vi "nanomsg_pub.vi"() -> ()   [LabVIEW 2014]
uses:
  lvnanomsg/nanomsg_context.lvclass
  lvnanomsg/nanomsg_socket.lvclass
panel:
  out "loop":i32=1
  in  "port":i32=5555
  # "Nanomsg publisher VI"
  # "Launch multiple instances of this template VI on different ports, and use zmq_sub.vit to subscribe to them all simultaneously."
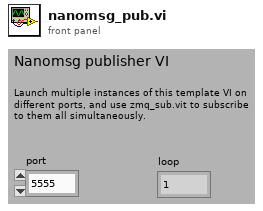
[diagram p1: front panel]
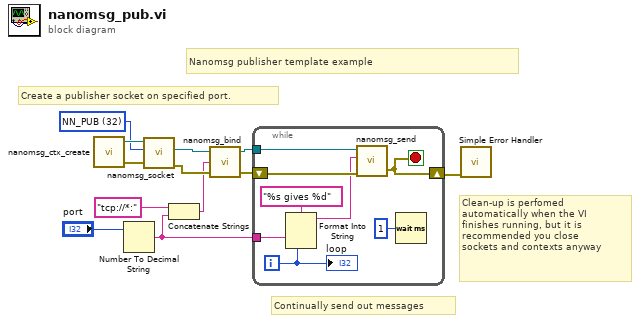
[diagram p0: block diagram]
diagram:
  w10 = 32 items=["NN_WS"=-4, "NN_TCP"=-3, "NN_IPC"=-2, "NN_INPROC"=-1, "NN_SOL_SOCKET"=0, "NN_PAIR"=16, "NN_PUB"=32, "NN_SUB"=33, "NN_REQ"=48, "NN_REP"=49, "NN_PUSH"=80, "NN_PULL"=81, "NN_SURVEYOR"=98, "NN_RESPONDENT"=99, "NN_BUS"=112] ("socket type")
  # "Clean-up is perfomed\nautomatically when the VI\nfinishes running, but it is\nrecommended you close\nsockets and contexts anyway"
  # "Nanomsg publisher template example"
  # "Continually send out messages"
  # "Create a publisher socket on specified port."
  n1 = call "nanomsg_ctx_create.vi"() -> ("error out"=w9:errorcluster, "context out"=w12:refnum<class "nanomsg_context.lvclass">)  [unwired: 4 in]
  n2 = Number To Decimal String(number="port") -> (decimal integer string=w2:string)  [unwired: 1 in]
  n3 = call "nanomsg_socket.vi"("error in"=w9, "socket type"=w10, "context in"=w12) -> ("error out"=w8:errorcluster, "socket out"=w1:refnum<class "nanomsg_socket.lvclass">)  [unwired: 2 in, 1 out]
  n4 = Concatenate Strings("tcp://*:" ("endpoint"), w2) -> (w4:string)
  n5 = call "nanomsg_bind.vi"("error in"=w8, "endpoint"=w4, "socket in"=w1) -> ("error out"=w6:errorcluster, "socket out"=w11:refnum<class "nanomsg_socket.lvclass">)  [unwired: 1 in]
  n6 = while {
    tunnel: w11 -> [w20]
    shift-right: [w15] -> w5
    shift-left: w6 -> [w19]
    tunnel: w2 -> [w14]
    i -> [w13]
    stop <- w15 stop-if-true
    n7 = Format Into String(format string="%s gives %d", w14, w13) -> (resulting string=w17:string)  [unwired: 2 in, 1 out]
    n8 = call "nanomsg_send.vi"("error in"=w19, "data"=w17, "socket in"=w20) -> ("error out"=w15:errorcluster)  [unwired: 1 in, 1 out]
    n9 = Wait (ms)(milliseconds to wait=u32 1) -> ()  [unwired: 1 out]
    "loop" <- w13
  }
  n10 = call <vilib>:"Simple Error Handler.vi"("error in (no error)"=w5) -> ()  [unwired: 4 in, 5 out]
